vi "histo_init@15.vi"(8 "Histo (e)":T1, 9 "Pièce":T2) -> (2 "Histo (s)":T1)   [LabVIEW 2010, in "lv_07.lvlib"]
uses:
  lv_07.lvlib
  c_pi_wilson.ctl
  c_histo.ctl
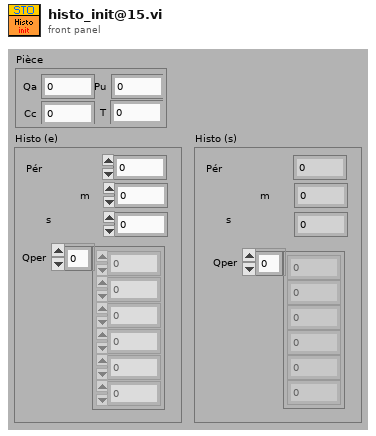
[diagram p1: front panel]
types:
  T1 = typedef "lv_07.lvlib/c_histo.ctl" = cluster{"Pér":dbl, "Qper":dbl[], "s":dbl, "m":dbl}
  T2 = typedef "lv_07.lvlib/c_pi_wilson.ctl" = cluster{"T":dbl, "Pu":dbl, "Qa":dbl, "Cc":dbl}
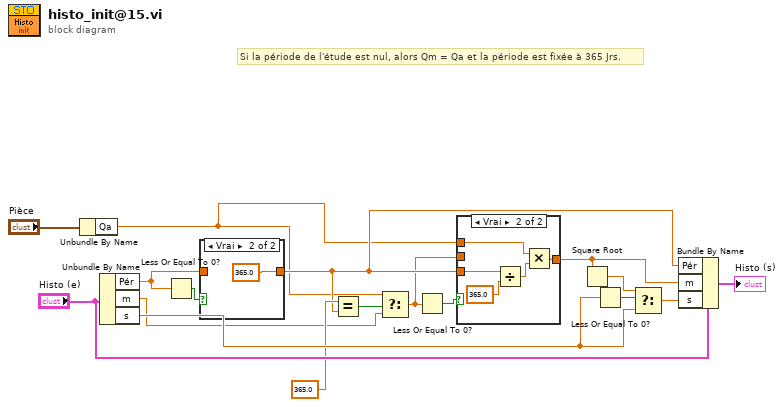
[diagram p0: block diagram]
diagram:
  # "Si la période de l'étude est nul, alors Qm = Qa et la période est fixée à 365 Jrs."
  n1 = Unbundle By Name("Pièce") -> ("Qa"=w1:dbl)
  n2 = Unbundle By Name("Histo (e)") -> ("Pér"=w7:dbl, "m"=w3:dbl, "s"=w11:dbl)
  n3 = Less Or Equal To 0?(x=w7) -> (x <= 0?=w16:bool)
  n4 = case shown="Vrai" w16 {
    tunnel: [w18 365.0] -> w4
    tunnel: w7 -> [w18 _]
    frame False {
    }
    frame True {
    }
  }
  n5 = Equal?(x=365.0, y=w4) -> (x = y?=w5:bool)
  n6 = Select(t=w1, s=w5, f=w3) -> (s? t:f=w2:dbl)
  n7 = Less Or Equal To 0?(x=w2) -> (x <= 0?=w12:bool)
  n8 = case shown="Vrai" w12 {
    tunnel: w4 -> [_ w25]
    tunnel: [w20 w22] -> w9
    tunnel: w2 -> [w20 _]
    tunnel: w1 -> [_ w21]
    frame False {
    }
    frame True {
      n9 = Divide(x=w25, y=365.0) -> (x/y=w23:dbl)
      n10 = Multiply(x=w21, y=w23) -> (x*y=w22:dbl)
    }
  }
  n11 = Square Root(x=w9) -> (sqrt(x)=w14:dbl)
  n12 = Less Or Equal To 0?(x=w11) -> (x <= 0?=w15:bool)
  n13 = Select(t=w14, s=w15, f=w11) -> (s? t:f=w13:dbl)
  n14 = Bundle By Name(cluster="Histo (e)", "Pér"=w4, "m"=w9, "s"=w13) -> (→"Histo (s)":T1)
